vi "ProcessJSONImmediateVariables.vi"(8 "error in (no error)":errorcluster, 10 "JSON Array":string) -> (0 "error out":errorcluster, 1 "JSON Error string":string, 2 "Variable Requested":i32, 3 "JSON Response String":string)   [LabVIEW 2013]
doc: "Extracts and valiadates the array of JSON Variables before entering them in the appropriate queue for processing. Generates an appropriate JSON response object."
uses:
  JSONVarSet.ctl
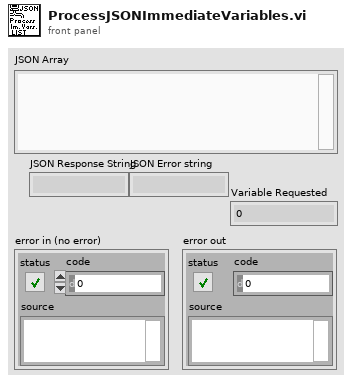
[diagram p1: front panel]
types:
  T1 = typedef "JSONVarSet.ctl" = string[]
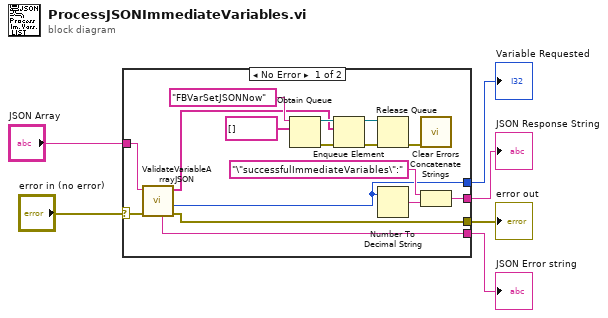
[diagram p0: block diagram]
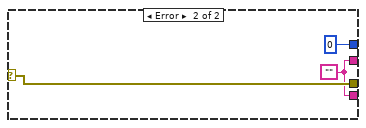
[diagram p2: hidden frame]
diagram:
  n1 = case shown="No Error" "error in (no error)" {
    selector: "error in (no error)" -> [w21 w25]
    tunnel: "JSON Array" -> [w22 _]
    tunnel: [w7 w25] -> w6
    tunnel: [w15 0 ("offset past token")] -> w4
    tunnel: [w19 w23] -> w3
    tunnel: [w16 w23] -> w2
    frame No Error {
      n2 = call "ValidateVariableArrayJSON.vi"("error in (no error)"=w21, "JSONVariableArray"=w22) -> ("error out"=w7:errorcluster, "Valid Count"=w15:i32, "JSONVarSet"=w12:T1, "JSONErrorResponse"=w19:string)  [unwired: 5 in, 1 out]
      n3 = Obtain Queue(name (unnamed)="FBVarSetJSONNow", element data type=T1 [] ("JSONVarSet")) -> (queue out=w13:refnum<queue>, error out=w14:errorcluster)  [unwired: 3 in, 1 out]
      n4 = Enqueue Element(queue=w13, element=w12, error in (no error)=w14) -> (queue out=w8:refnum<queue>, error out=w9:errorcluster)  [unwired: 1 in, 1 out]
      n5 = Release Queue(queue=w8, error in (no error)=w9) -> (error out=w10:errorcluster)  [unwired: 1 in, 2 out]
      n6 = Number To Decimal String(number=w15) -> (decimal integer string=w18:string)  [unwired: 1 in]
      n7 = call <vilib>:"Clear Errors.vi"("error in (no error)"=w10) -> ()  [unwired: 6 in, 1 out]
      n8 = Concatenate Strings("\"successfulImmediateVariables\":" ("string"), w18) -> (w16:string)
    }
    frame Error {
      w23 = ""
    }
  }
  "error out" <- w6
  "Variable Requested" <- w4
  "JSON Error string" <- w3
  "JSON Response String" <- w2
